vi "LVIS_DeleteLastMeas.vi"(8 "Error In":errorcluster) -> (0 "Error Out":errorcluster)   [LabVIEW 2015]
doc: "Determines the Measurement Info based on the LVIS_Settings file and passed in values, giving precedence to the file and deriving values where requested."
uses:
  Globals/LVIS_IsGlobal.vi
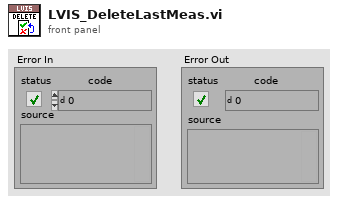
[diagram p1: front panel]
types:
  T1 = cluster{"EventInfo":cluster{"EventName":string, "EventStart":string, "EventStop":string, "EventStatus":string, "EventClientID":string, "IS_EventID":string, "EventMeta":string, "ProductLine":string, "ProcessName":string, "Station":string, "Operator":string, "SN":string, "Model":string, "Manufacturer":string}, "TestInfo":cluster{"TestName":string, "TestDateTime":string, "TestStatus":string, "TestClientID":string, "IS_TestID":string, "TestMeta":string}, "MeasInfo":cluster{"MeasName":string, "MeasDateTime":string, "MeasStatus":string, "MeasClientID":string, "IS_MeasID":string, "MeasMeta":string, "MeasType":string, "MeasValue":string, "LL":string, "LL Comp":string, "HL":string, "HL Comp":string, "Units":string}}[]
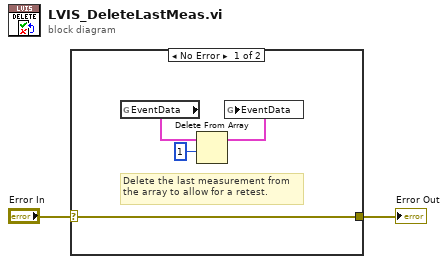
[diagram p0: block diagram]
diagram:
  n1 = case shown="No Error" "Error In" {
    selector: "Error In" -> [w3 w7]
    tunnel: [w3 w7] -> w1
    frame No Error {
      # "Delete the last measurement from\nthe array to allow for a retest."
      n2 = global read "LVIS_IsGlobal.vi" "EventData"() -> (w4:T1)
      n3 = Delete From Array(array=w4, length=1) -> (array with subset deleted=w6:T1)  [unwired: 1 in, 1 out]
      n4 = global write "LVIS_IsGlobal.vi" "EventData"(w6) -> ()
    }
    frame Error {
    }
  }
  "Error Out" <- w1
